vi "WH and AH initialization.vi"(8 "error in (no error)":errorcluster, 10 "Dynamic Data":dynamicdata(graph), 11 "Universal Power Meter.lvlib:Universal Card.lvclass":refnum<class "Universal Card.lvclass">) -> (0 "error out":errorcluster, 3 "Universal Power Meter.lvlib:Universal Card.lvclass 2":refnum<class "Universal Card.lvclass">)   [LabVIEW 2013, in "Universal Power Meter.lvlib" / "Universal Card.lvclass"]
uses:
  Universal Card.lvclass
  Universal Card.lvclass/Universal Card.ctl
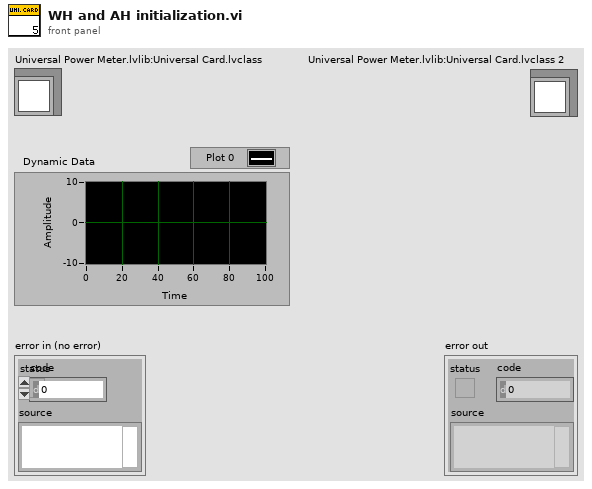
[diagram p1: front panel]
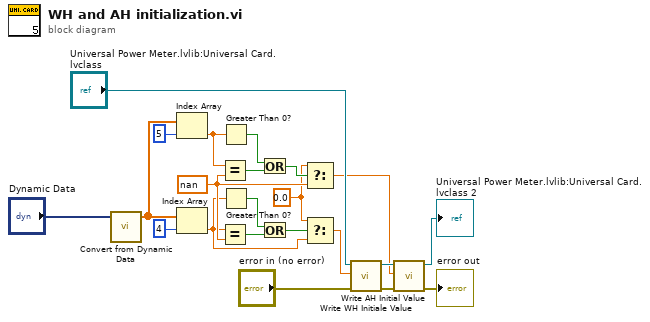
[diagram p0: block diagram]
diagram:
  w12 = 0.0 ("t")
  w13 = nan
  n1 = call "Convert from Dynamic Data"("Dynamic Data Type"="Dynamic Data") -> ("Array"=w3:dbl[])  [unwired: 3 in]
  n2 = Index Array(array=w3, index=5) -> (element=w1:dbl)
  n3 = Index Array(array=w3, index=4) -> (element=w4:dbl)
  n4 = Equal?(x=w1, y=w13) -> (x = y?=w16:bool)
  n5 = Equal?(x=w4, y=w13) -> (x = y?=w17:bool)
  n6 = Greater Than 0?(x=w1) -> (x > 0?=w18:bool)
  n7 = Greater Than 0?(x=w4) -> (x > 0?=w19:bool)
  n8 = Or(x=w18, y=w16) -> (x .or. y?=w14:bool)
  n9 = Or(x=w19, y=w17) -> (x .or. y?=w15:bool)
  n10 = Select(t=w12, s=w14, f=w13) -> (s? t:f=w10:dbl)
  n11 = Select(t=w12, s=w15, f=w4) -> (s? t:f=w11:dbl)
  n12 = call "Write WH Initiale Value.vi"("error in (no error)"="error in (no error)", "WH Initiale Value"=w11, "Universal Card in"="Universal Power Meter.lvlib:Universal Card.lvclass") -> ("error out"=w7:errorcluster, "Universal Card out"=w22:refnum<class "Universal Card.lvclass">)  [unwired: 7 in]
  n13 = call "Write AH Initial Value.vi"("error in (no error)"=w7, "AH Initial Value"=w10, "Universal Card in"=w22) -> ("error out"=→"error out":errorcluster, "Universal Card out"=→"Universal Power Meter.lvlib:Universal Card.lvclass 2":refnum<class "Universal Card.lvclass">)  [unwired: 7 in]
